vi "GetFitValues.vi"(8 "error in (no error)":errorcluster, 11 "Exponential Fit in":refnum<class "Exponential Fit.lvclass">) -> (0 "error out":errorcluster, 1 "Response Parameters":T1, 2 "Stimulus Parameters":T1, 3 "Exponential Fit out":refnum<class "Exponential Fit.lvclass">)   [LabVIEW 2013, in "Exponential Fit.lvclass"]
uses:
  Exponential Fit.lvclass
  Exponential Fit Parameters.ctl
  Exponential Fit.lvclass/Exponential Fit.ctl
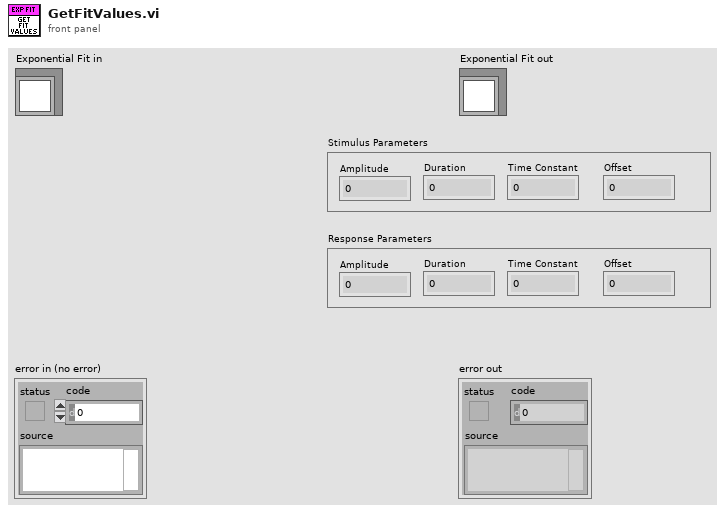
[diagram p1: front panel]
types:
  T1 = typedef "Exponential Fit.lvclass/Exponential Fit Parameters.ctl" = cluster{"Amplitude":dbl, "Duration":dbl, "Time Constant":dbl, "Offset":dbl}
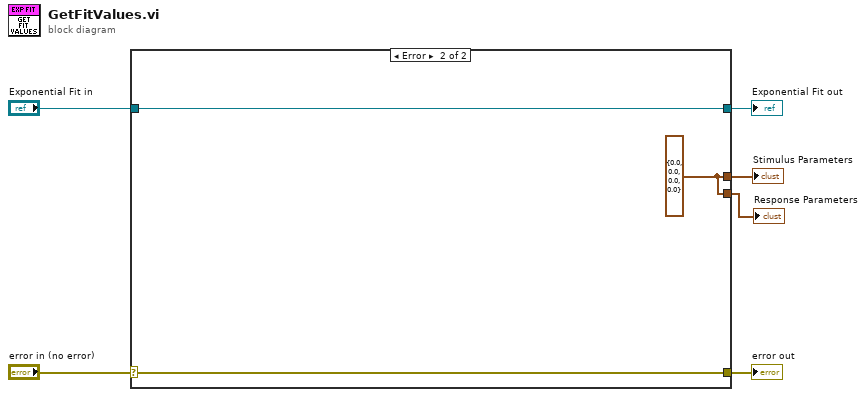
[diagram p0: block diagram]
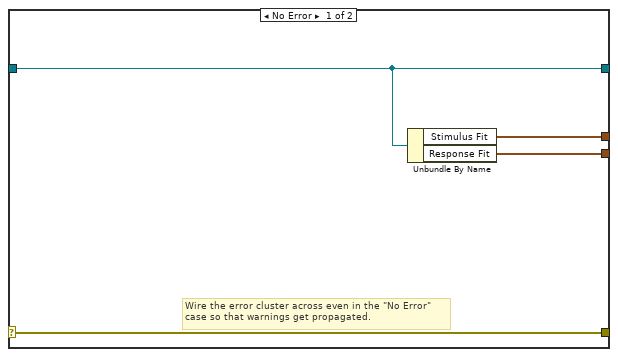
[diagram p2: hidden frame]
diagram:
  n1 = case shown="Error" "error in (no error)" {
    selector: "error in (no error)" -> [w10 w13]
    tunnel: [w10 w13] -> w5
    tunnel: [w9 w12] -> w3
    tunnel: "Exponential Fit in" -> [w9 w12]
    tunnel: [w8 w11] -> w2
    tunnel: [w7 w11] -> w1
    frame No Error {
      # "Wire the error cluster across even in the \"No Error\"\ncase so that warnings get propagated."
      n2 = Unbundle By Name(w9) -> ("Stimulus Fit"=w8:T1, "Response Fit"=w7:T1)
    }
    frame Error {
      w11 = T1 {"Amplitude"=0.0, "Duration"=0.0, "Time Constant"=0.0, "Offset"=0.0} ("Stimulus Fit")
    }
  }
  "error out" <- w5
  "Exponential Fit out" <- w3
  "Stimulus Parameters" <- w2
  "Response Parameters" <- w1
